vi "Compose LabVIEW Object - String - Value.vi"() -> ()   [LabVIEW 2017, in "Composition.Tests.lvlib"]
uses:
  Composition.Tests.lvlib
  92f102a0-c856-46da-bf7d-d489e92c860f.vi
  Classes/String/String.lvclass
  <vilib>/addons/_JKI Toolkits/Caraya/classes/Assert/Assert.lvclass
  <vilib>/addons/_JKI Toolkits/Caraya/classes/Test/Test.lvclass
panel:
  out "error out":errorcluster
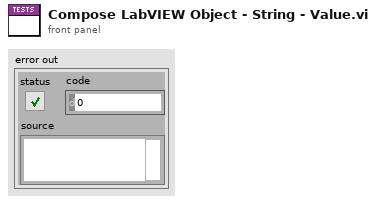
[diagram p1: front panel]
types:
  T1 = cluster{"Major":u16, "Minor":u16, "Fix":u16, "Build":u16}[]
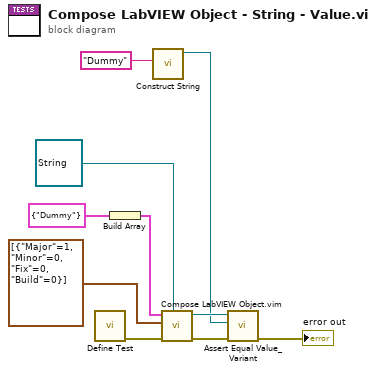
[diagram p0: block diagram]
diagram:
  n1 = call <vilib>:"Define Test.vi"() -> ("error out"=w1:errorcluster)  [unwired: 11 in]
  n2 = Build Array(cluster{string} {"Dummy"}) -> (w6:cluster{string}[])
  n3 = call "Construct String.vi"("String"="Dummy") -> ("String out"=w2:refnum<class "String.lvclass">)  [unwired: 9 in, 1 out]
  n4 = call "Compose LabVIEW Object.vim"("Type"=refnum<class "String.lvclass"> refnum ("Reflection.Tests.lvlib:String.lvclass"), "error in (no error)"=w1, "Library Versions"=T1 [{"Major"=1, "Minor"=0, "Fix"=0, "Build"=0}], "Private Data Clusters"=w6) -> ("error out"=w5:errorcluster, "LabVIEW Object"=w3:refnum<class "String.lvclass">)  [unwired: 6 in]
  n5 = call <vilib>:"Assert Equal Value_Variant.vi"("error in (no error)"=w5, "Y"=w2, "X"=w3) -> ("error out"=→"error out":errorcluster)  [unwired: 8 in]
